vi "Untitled 4.vi"() -> ()   [LabVIEW 2015]
uses:
  Interlocks/Interlock Bool/Interlock Bool.lvclass
  Interlocks/Interlock DBL/Range/Interlock Range.lvclass
  Interlocks/Interlock/Interlock.lvclass
  Interlocks/Interlock DBL/Range/Interlock Range.lvclass/Interlock Range.ctl
  Interlocks/Interlock Bool/Interlock Bool.lvclass/Interlock Bool.ctl
panel:
  out "Interlock out":bool
  out "Array":errorcluster[](array[cluster])
  in  "SHV":refnum<k21>="ni.var.psp://10.2.0.20/AMS Gas SHV/Gauges/Baratron 1"
  in  "shared variable refnum in":refnum<k21>="ni.var.psp://10.2.0.20/AMS Gas SHV/Stepper/HOME Switch"
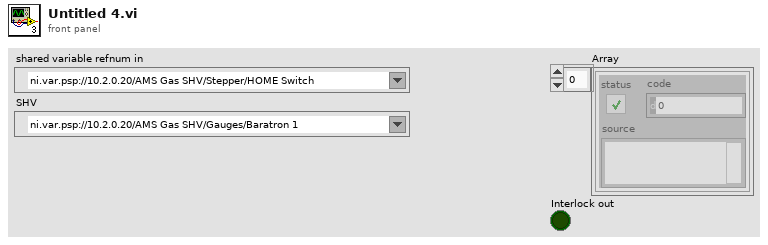
[diagram p1: front panel]
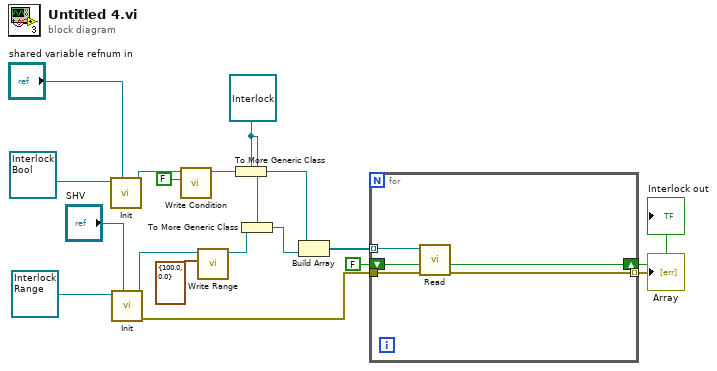
[diagram p0: block diagram]
diagram:
  w3 = refnum<class "Interlock.lvclass"> refnum ("Interlock.lvclass")
  n1 = call-dynamic "Init.vi"("SHV"="shared variable refnum in", "Interlock in"=refnum<class "Interlock Bool.lvclass"> refnum ("Interlock Bool.lvclass")) -> ("Interlock out"=w17:refnum<class "Interlock Bool.lvclass">)  [unwired: 8 in, 1 out]
  n2 = call-dynamic "Init.vi"("SHV"="SHV", "Interlock in"=refnum<class "Interlock Range.lvclass"> refnum ("Interlock DBL.lvclass")) -> ("error out"=w8:errorcluster, "Interlock out"=w12:refnum<class "Interlock Range.lvclass">)  [unwired: 8 in]
  n3 = call "Write Condition.vi"("Interlock Condition"=FALSE, "Interlock Bool in"=w17) -> ("Interlock Bool out"=w10:refnum<class "Interlock Bool.lvclass">)  [unwired: 8 in, 1 out]
  n4 = call "Write Range.vi"("Range"=cluster{"Upper Limit":dbl, "Lower Limit":dbl} {"Upper Limit"=100.0, "Lower Limit"=0.0}, "Interlock Bool in"=w12) -> ("Interlock Bool out"=w2:refnum<class "Interlock Range.lvclass">)  [unwired: 8 in, 1 out]
  n5 = To More Generic Class(target class=w3, reference=w10) -> (generic class reference=w4:refnum<class "Interlock.lvclass">)
  n6 = To More Generic Class(target class=w3, reference=w2) -> (generic class reference=w1:refnum<class "Interlock.lvclass">)
  n7 = Build Array(w4, w1) -> (w9:refnum<class "Interlock.lvclass">[])
  n8 = for {
    tunnel: w9 -> [w23] mode=indexing
    tunnel: w8 -> [w22]
    shift-right: [w21] -> w5
    shift-left: FALSE ("Interlock out") -> [w20]
    tunnel: [w19] -> w6 mode=indexing
    n9 = call-dynamic "Read.vi"("error in (no error)"=w22, 9:"Interlock in"=w20, 11:"Interlock in"=w23) -> ("error out"=w19:errorcluster, "Interlock out"=w21:bool)  [unwired: 4 in, 3 out]
  }
  "Array" <- w6
  "Interlock out" <- w5
